vi "Read Serializer.vi"(11 "ConfigManager in":refnum<class "ConfigManager.lvclass">) -> (2 "Serializer":refnum<class "Serializer.lvclass">, 3 "ConfigManager out":refnum<class "ConfigManager.lvclass">)   [LabVIEW 2013, in "CfgManager.lvlib" / "ConfigManager.lvclass"]
uses:
  ConfigManager.lvclass
  <vilib>/LabVIEW Open Source Project/Serializer/Serializer/Serializer.lvclass
  ConfigManager.lvclass/ConfigManager.ctl
  <vilib>/LabVIEW Open Source Project/Serializer/Serializer.PlainText/Serializer.PlainText.lvclass
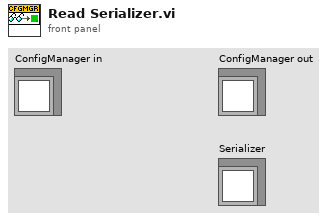
[diagram p1: front panel]
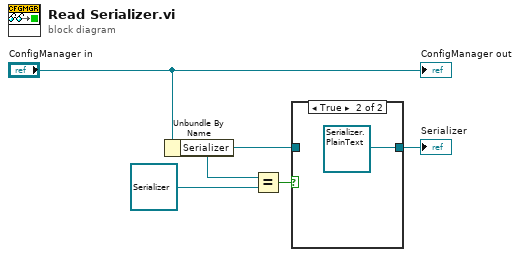
[diagram p0: block diagram]
diagram:
  n1 = Unbundle By Name("ConfigManager in") -> ("Serializer"=w2:refnum<class "Serializer.lvclass">)
  n2 = Equal?(x=w2, y=refnum<class "Serializer.lvclass"> refnum) -> (x = y?=w3:bool)
  n3 = case shown="True" w3 {
    tunnel: w2 -> [w6 _]
    tunnel: [w6 refnum<class "Serializer.PlainText.lvclass"> refnum ("Serializer.PlainText.lvclass")] -> w1
    frame False {
    }
    frame True {
    }
  }
  "Serializer" <- w1
  "ConfigManager out" <- "ConfigManager in"
